vi "AddAlarmMeasurement.vi"(6 "OID Numbers":string[](array[string]), 7 "Model Information":string[][](array[string]), 8 "Error In":errorcluster, 11 "Measurements To Read Array In":u16[](array[numeric])) -> (0 "Error Out":errorcluster, 3 "Measurements To Read Array Out":u16[](array[numeric]))   [LabVIEW 2018, in "SensorPlugins.lvlib" / "RoomAlert.lvclass"]
doc: "Adds an alarm measurement to ensure the RoomAlert plugin is always checking if an alarm occured."
uses:
  RoomAlert.lvclass
  <vilib>/Utility/error.llb/Error Cluster From Error Code.vi
  <vilib>/ErrorRing/Error Ring.xnode
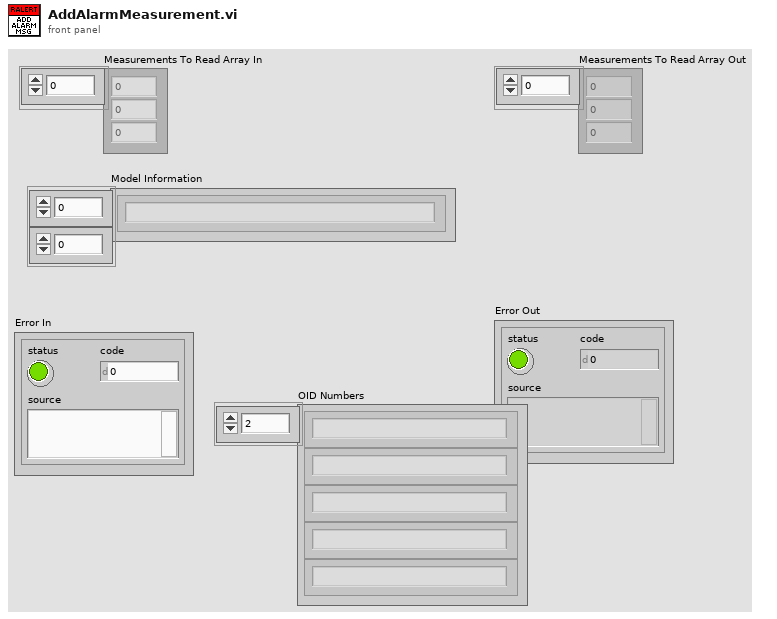
[diagram p1: front panel]
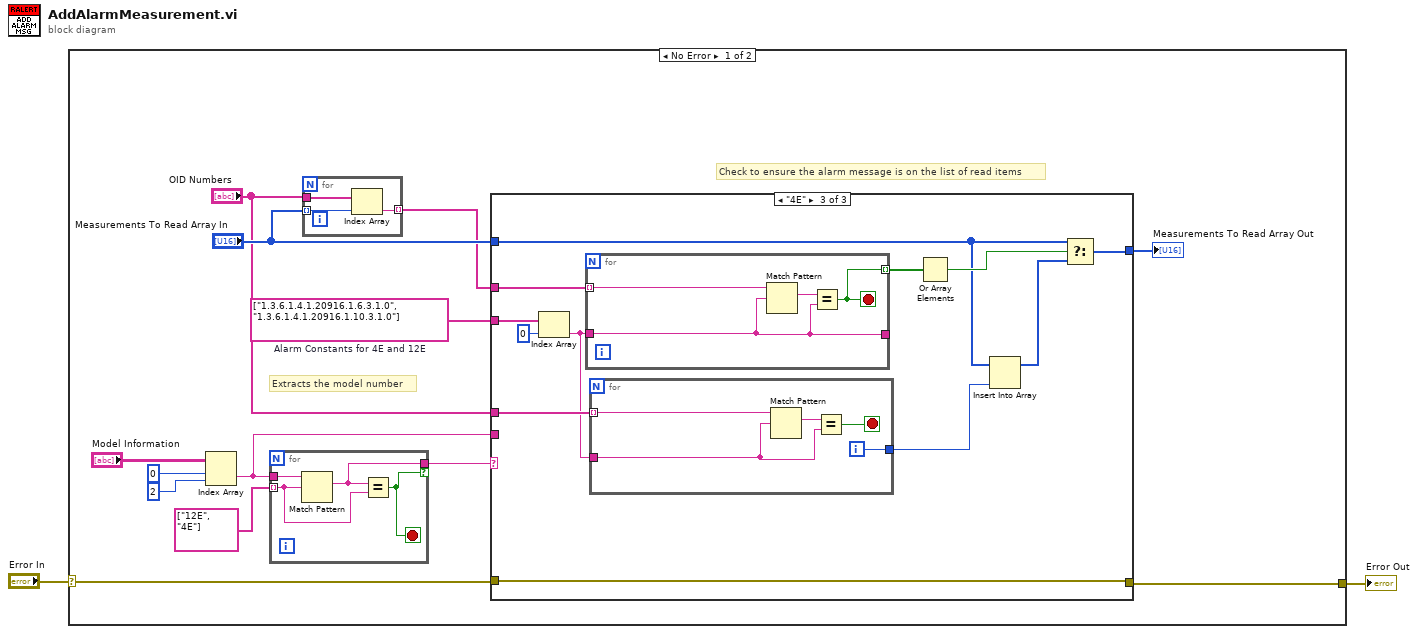
[diagram p0: block diagram]
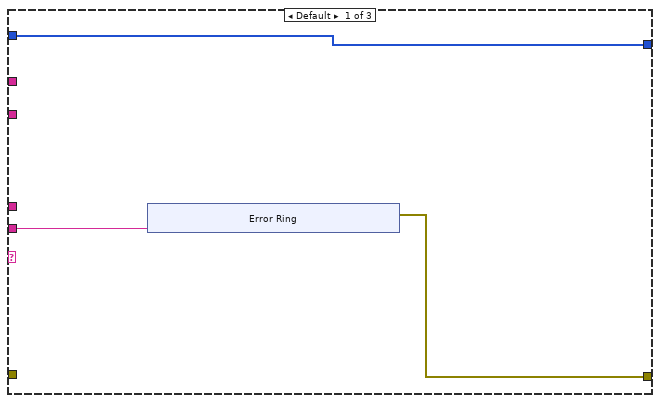
[diagram p2: hidden frame]
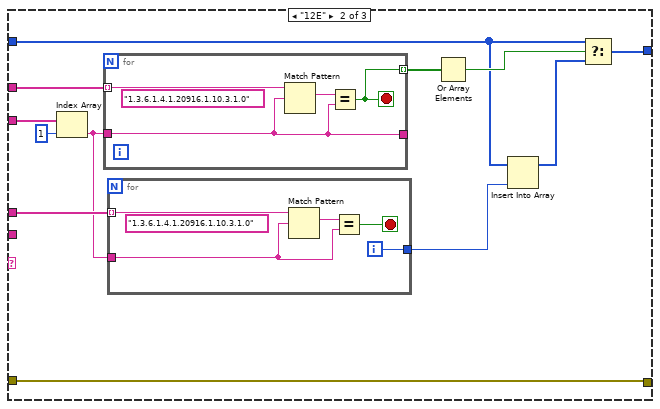
[diagram p3: hidden frame]
diagram:
  n1 = case shown="No Error" "Error In" {
    selector: "Error In" -> [w11 w75]
    tunnel: [w10 w75] -> w1
    frame No Error {
      w3 = string[] ["1.3.6.1.4.1.20916.1.6.3.1.0", "1.3.6.1.4.1.20916.1.10.3.1.0"]  # Alarm Constants for 4E and 12E
      # "Extracts the model number"
      # "Check to ensure the alarm message is on the list of read items"
      n2 = Index Array(array="Model Information", index (row)=0, index (col)=2 ("disabled index (col)")) -> (element=w4:string)
      n3 = for {
        tunnel: w4 -> [w19]
        tunnel: string[] ["12E", "4E"] -> [w18] mode=indexing
        tunnel: [w17] -> w5 if=w16
        stop <- w16 stop-if-true
        n4 = Match Pattern(string=w19, regular expression=w18) -> (match substring=w17:string)  [unwired: 1 in, 3 out]
        n5 = Equal?(x=w17, y=w18) -> (x = y?=w16:bool)
      }
      n6 = for {
        tunnel: "Measurements To Read Array In" -> [w21] mode=indexing
        tunnel: "OID Numbers" -> [w22]
        tunnel: [w20] -> w8 mode=indexing
        n7 = Index Array(array=w22, index=w21) -> (element=w20:string)
      }
      n8 = case shown="\"4E\"" w5 {
        tunnel: "Measurements To Read Array In" -> [w25 w38 w59]
        tunnel: [w25 w40 w61] -> w15
        tunnel: w11 -> [_ w44 w65]
        tunnel: [w24 w44 w65] -> w10
        tunnel: w8 -> [_ w43 w64]
        tunnel: "OID Numbers" -> [_ w39 w60]
        tunnel: w4 -> [w23 _ _]
        tunnel: w3 -> [_ w35 w56]
        frame Default {
          n9 = xnode "Error Ring"("parameter 0"=w23) -> ("error out"=w24:errorcluster)
        }
        frame "12E" {
          n10 = Index Array(array=w35, index=1) -> (element=w34:string)
          n11 = for {
            tunnel: w43 -> [w53] mode=indexing
            tunnel: [w51] -> w42 mode=indexing
            tunnel: [w50] -> _
            tunnel: w34 -> [w50]
            stop <- w51 stop-if-true
            (unwired) "1.3.6.1.4.1.20916.1.10.3.1.0" ("regular expression")
            n12 = Match Pattern(string=w53, regular expression=w50) -> (match substring=w52:string)  [unwired: 1 in, 3 out]
            n13 = Equal?(x=w52, y=w50) -> (x = y?=w51:bool)
          }
          n14 = for {
            tunnel: w39 -> [w49] mode=indexing
            tunnel: [w46] -> w37
            tunnel: w34 -> [w45]
            i -> [w46]
            stop <- w47 stop-if-true
            (unwired) "1.3.6.1.4.1.20916.1.10.3.1.0" ("regular expression")
            n15 = Match Pattern(string=w49, regular expression=w45) -> (match substring=w48:string)  [unwired: 1 in, 3 out]
            n16 = Equal?(x=w48, y=w45) -> (x = y?=w47:bool)
          }
          n17 = Or Array Elements(Boolean array=w42) -> (logical OR=w41:bool)
          n18 = Insert Into Array(array=w38, new element=w37) -> (w36:u16[])  [unwired: 1 in]
          n19 = Select(t=w38, s=w41, f=w36) -> (s? t:f=w40:u16[])
        }
        frame "4E" {
          n20 = Index Array(array=w56, index=0) -> (element=w55:string)
          n21 = for {
            tunnel: w64 -> [w74] mode=indexing
            tunnel: [w72] -> w63 mode=indexing
            tunnel: [w71] -> _
            tunnel: w55 -> [w71]
            stop <- w72 stop-if-true
            n22 = Match Pattern(string=w74, regular expression=w71) -> (match substring=w73:string)  [unwired: 1 in, 3 out]
            n23 = Equal?(x=w73, y=w71) -> (x = y?=w72:bool)
          }
          n24 = for {
            tunnel: w60 -> [w70] mode=indexing
            tunnel: [w67] -> w58
            tunnel: w55 -> [w66]
            i -> [w67]
            stop <- w68 stop-if-true
            n25 = Match Pattern(string=w70, regular expression=w66) -> (match substring=w69:string)  [unwired: 1 in, 3 out]
            n26 = Equal?(x=w69, y=w66) -> (x = y?=w68:bool)
          }
          n27 = Or Array Elements(Boolean array=w63) -> (logical OR=w62:bool)
          n28 = Insert Into Array(array=w59, new element=w58) -> (w57:u16[])  [unwired: 1 in]
          n29 = Select(t=w59, s=w62, f=w57) -> (s? t:f=w61:u16[])
        }
      }
      "Measurements To Read Array Out" <- w15
    }
    frame Error {
    }
  }
  "Error Out" <- w1
